vi "Claw Grab Activate.vi"(9 "Let Go":bool, 11 "Grab":bool) -> ()   [LabVIEW 2012]
uses:
  <vilib>/Rock Robotics/WPI/Solenoid/WPI_SolenoidValue.ctl
  <vilib>/Rock Robotics/WPI/Solenoid/WPI_SolenoidSetEnum.vi
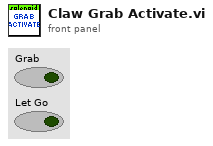
[diagram p1: front panel]
types:
  T1 = typedef "WPI_SolenoidValue.ctl" = enum16{"Off", "On", "Forward", "Reverse"}
  T2 = typedef "WPI_SolenoidDevRef.ctl" = cluster{"DevStatus":errorcluster, "Solenoid Module":T3, "Forward Solenoid Channel":T4, "Reverse Solenoid Channel":T4}
  T3 = typedef "FPGA_TypedefSolenoidModule.ctl" = enum16{"Solenoid Module 1", "Solenoid Module 2"}
  T4 = typedef "WPI_SolenoidChannel.ctl" = enum8{"Solenoid 1", "Solenoid 2", "Solenoid 3", "Solenoid 4", "Solenoid 5", "Solenoid 6", "Solenoid 7", "Solenoid 8", "Invalid"}
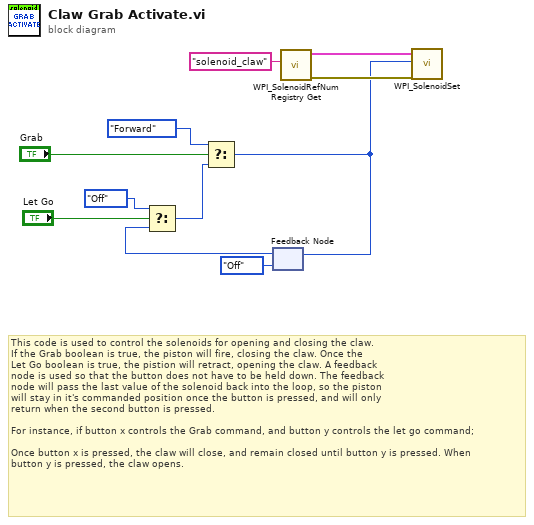
[diagram p0: block diagram]
diagram:
  # "This code is used to control the solenoids for opening and closing the claw.\nIf the Grab boolean is true, the piston will fire, closing the claw. Once the \nLet Go boolean is true, the pistion will retract, opening the claw. A feedback\nnode is used so that the button does not have to be held down. The feedback\nnode will pass the last value of the solenoid back into the loop, so the piston \nwill stay in it's commanded position once the button is pressed, and will only \nreturn when the second button is pressed. \n\nFor instance, if button x controls the Grab command, and button y controls the let go command; \n\nOnce button x is pressed, the claw will close, and remain closed until button y is pressed. When \nbutton y is pressed, the claw opens."
  n1 = feedback #1(WPI_SolenoidValue."Off" ("Value")) -> (w2:T1)
  n2 = Select(t=WPI_SolenoidValue."Off" ("Value"), s="Let Go", f=w2) -> (s? t:f=w4:T1)
  n3 = Select(t=WPI_SolenoidValue."Forward" ("Value"), s="Grab", f=w4) -> (s? t:f=w3:T1)
  n4 = feedback-in #1(w3) -> ()
  n5 = call <vilib>:"WPI_SolenoidRefNum Registry Get.vi"("refnum name"="solenoid_claw") -> ("error out"=w10:errorcluster, "SolenoidDevRef"=w11:T2)  [unwired: 9 in]
  n6 = call-poly <vilib>:"WPI_SolenoidSet.vi"("error in (no error)"=w10, "Value"=w3, "SolenoidDevRef"=w11) -> ()  [unwired: 7 in, 2 out]
